vi "SetCalcParams.vi"(8 "error in":errorcluster, 9 "Experiment.lvclass":refnum<class "Experiment.lvclass">, 11 "Interface.lvclass":refnum<class "Interface.lvclass">) -> (0 "error out":errorcluster, 1 "Experiment.lvclass Out":refnum<class "Experiment.lvclass">, 3 "Interface.lvclass Out":refnum<class "Interface.lvclass">)   [LabVIEW 2019, in "Interface.lvclass"]
doc: "Ce Vi prend les données d'acquisition et les formatte en tableau de \"string\" pour ensuite les sauvegarder sous le format .txt"
uses:
  Interface.lvclass
  Experiment Class/Experiment.lvclass
  Interface.lvclass/Interface.ctl
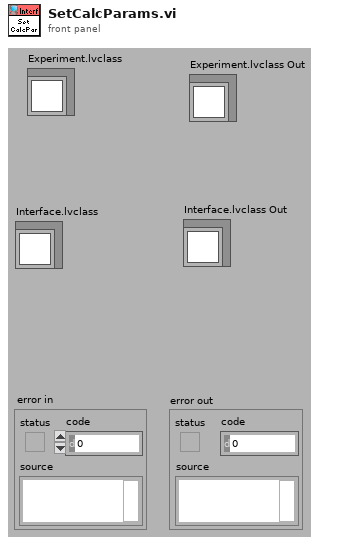
[diagram p1: front panel]
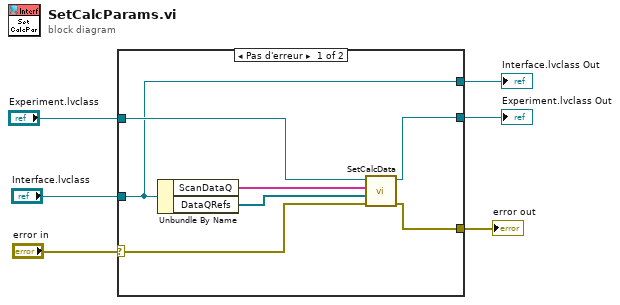
[diagram p0: block diagram]
diagram:
  n1 = case shown="Pas d'erreur" "error in" {
    selector: "error in" -> [w10 w16]
    tunnel: [w8 w16] -> w6
    tunnel: [w7 w15] -> w3
    tunnel: "Interface.lvclass" -> [w7 w15]
    tunnel: "Experiment.lvclass" -> [w11 w14]
    tunnel: [w9 w14] -> w1
    frame No Error {
      n2 = Unbundle By Name(w7) -> ("ScanDataQ"=w12:string[], "DataQRefs"=w13:refnum<queue>[])
      n3 = call "SetCalcData.vi"("error in (no error)"=w10, "DataQRefs"=w13, "ScanDataQ"=w12, "Experiment en entrée"=w11) -> ("error out"=w8:errorcluster, "Experiment en sortie"=w9:refnum<class "Experiment.lvclass">)  [unwired: 6 in]
    }
    frame Error {
    }
  }
  "error out" <- w6
  "Interface.lvclass Out" <- w3
  "Experiment.lvclass Out" <- w1
